vi "Set Switch Heater.vi"(2 "error in":T1, 3 "Switch Heater Control":bool, 4 "VISA resource name":refnum<visa-resource-name>) -> (0 "error out":T1, 1 "VISA resource name out":refnum<visa-resource-name>)   [LabVIEW 2019]
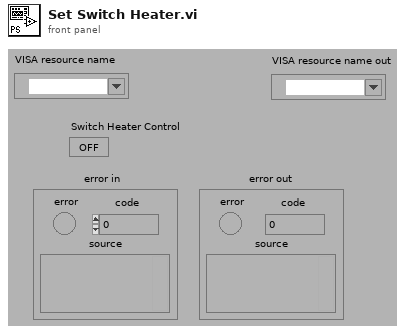
[diagram p1: front panel]
types:
  T1 = cluster{"error":bool, "code":i32, "source":string}
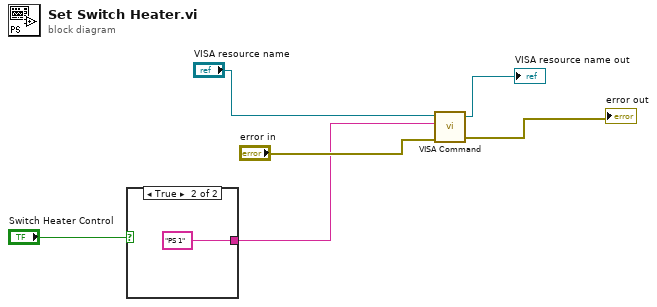
[diagram p0: block diagram]
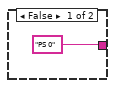
[diagram p2: hidden frame]
diagram:
  n1 = case shown="True" "Switch Heater Control" {
    tunnel: ["PS 0" "PS 1"] -> w3
    frame False {
    }
    frame True {
    }
  }
  n2 = call "VISA Command.vi"("error in (no error)"="error in", "Command"=w3, "VISA resource name"="VISA resource name") -> ("error out"=→"error out":errorcluster, "VISA resource name out"=→"VISA resource name out":refnum<visa-resource-name>)  [unwired: 1 in, 1 out]
